vi "Initialize Custom Device.vi"(8 "error in":errorcluster, 11 "custom device":T1=18446744073709551615 format="%.0x") -> (0 "error out":errorcluster, 3 "custom device out":T1 format="%.0x")   [LabVIEW 2020, in "AIM MIL-STD-1553 Scripting.lvlib"]
doc: "Adds Configuration File Section and Logging Section to the <b>custom device</b>."
uses:
  AIM MIL-STD-1553 Scripting.lvlib
  <vilib>/NI VeriStand/Custom Device API/Custom Device Item Ref.ctl
  <vilib>/NI VeriStand/Custom Device API/Custom Device API.lvlib
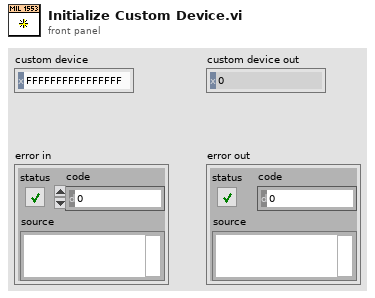
[diagram p1: front panel]
types:
  T1 = typedef "Custom Device API.lvlib/Custom Device Item Ref.ctl" = u64
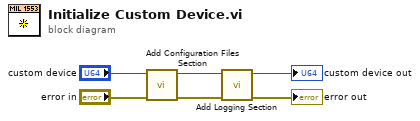
[diagram p0: block diagram]
diagram:
  n1 = call "Add Configuration Files Section.vi"("error in"="error in", "custom device"="custom device") -> ("error out"=w3:errorcluster, "custom device out"=w4:T1)  [unwired: 7 in, 1 out]
  n2 = call "Add Logging Section.vi"("error in"=w3, "Ballard MIL-STD 1553 custom device in"=w4) -> ("error out"=→"error out":errorcluster, "Ballard MIL-STD 1553 custom device out"=→"custom device out":T1)  [unwired: 7 in, 1 out]
